vi "Maui 2.0. Set Subpanels.Config.vi"(6 "Append (F)":bool, 8 "error in":errorcluster, 9 "Section Cluster":variant, 10 "Path":path, 11 "Maui 2.0 in":refnum<class "Maui 2.0.lvclass">) -> (0 "error out":errorcluster, 1 "Found?":bool, 2 "Subpanels":refnum<class "SMO.lvclass">[](array[class]), 3 "Maui 2.0 out":refnum<class "Maui 2.0.lvclass">)   [LabVIEW 2019, in "Maui 2.0.lvclass"]
uses:
  Maui 2.0.lvclass
  Typedefs/Maui 2.0/Maui 2.0 Configuration.ctl
  <vilib>/Utility/config.llb/NI_LVConfig.lvlib
  <vilib>/JKI/JKI SMO/SMO/SMO.lvclass
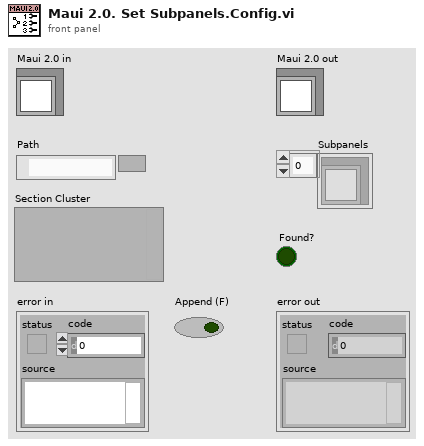
[diagram p1: front panel]
types:
  T1 = typedef "Maui 2.0.lvclass/Maui 2.0 Configuration.ctl" = cluster{"Paths":path[]}
  T2 = typedef "NI_LVConfig.lvlib/Config Data RefNum.ctl" = refnum<k1>
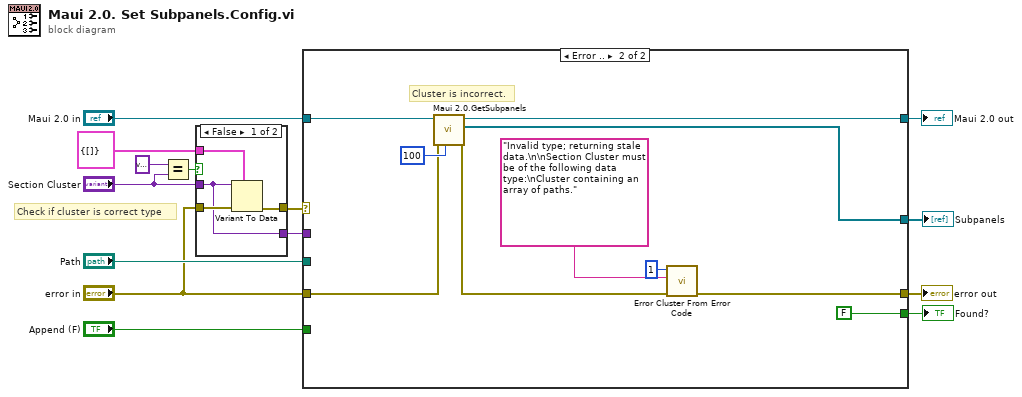
[diagram p0: block diagram]
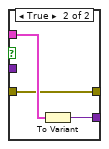
[diagram p2: hidden frame]
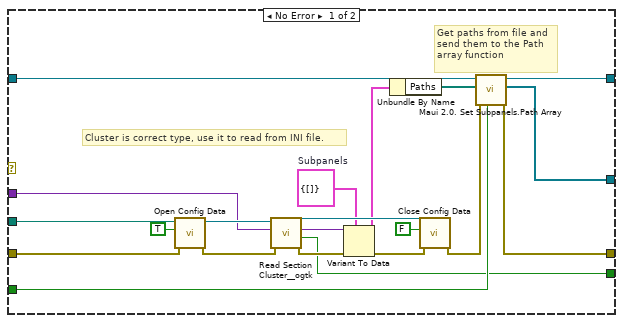
[diagram p3: hidden frame]
diagram:
  # "Check if cluster is correct type"
  n1 = Equal?(x=variant, y="Section Cluster") -> (x = y?=w3:bool)
  n2 = case shown="False" w3 {
    tunnel: T1 {"Paths"=[]} ("Subpanels") -> [w16 w21]
    tunnel: "Section Cluster" -> [w15 _]
    tunnel: [w18 w19] -> w6
    tunnel: "error in" -> [w17 w19]
    tunnel: [w15 w20] -> w5
    frame False {
      n3 = Variant To Data(error in=w17, type=w16, Variant=w15) -> (error out=w18:errorcluster)  [unwired: 1 out]
    }
    frame True {
      n4 = To Variant(anything=w21) -> (Variant=w20:variant)
    }
  }
  n5 = case shown="Error .." w6 {
    tunnel: "Path" -> [w42 _]
    tunnel: "error in" -> [w38 w43]
    tunnel: "Maui 2.0 in" -> [w32 w50]
    tunnel: [w31 w51] -> w12
    tunnel: [w29 w47] -> w11
    tunnel: "Append (F)" -> [w28 _]
    tunnel: [w25 w48] -> w9
    tunnel: [w24 FALSE ("all found?")] -> w8
    tunnel: w5 -> [w23 _]
    frame No Error {
      w22 = T1 {"Paths"=[]}  # Subpanels
      # "Get paths from file and send them to the Path array function"
      # "Cluster is correct type, use it to read from INI file."
      n6 = call <vilib>:"Open Config Data.vi"("error in (no error)"=w38, "create file if necessary (T)"=TRUE, "configuration file path"=w42) -> ("error out"=w37:errorcluster, "refnum"=w41:T2)  [unwired: 6 in, 1 out]
      n7 = call <userlib>:"Read Section Cluster__ogtk.vi"("error in (no error)"=w37, "Section Formatted Cluster Type"=w23, "refnum"=w41) -> ("error out"=w36:errorcluster, "all found?"=w24:bool, "Section Formatted Cluster"=w39:variant, "dup refnum"=w40:T2)  [unwired: 4 in, 1 out]
      n8 = Variant To Data(error in=w36, type=w22, Variant=w39) -> (data=w26:T1, error out=w35:errorcluster)
      n9 = Unbundle By Name(w26) -> ("Paths"=w27:path[])
      n10 = call <vilib>:"Close Config Data.vi"("error in (no error)"=w35, "write file if changed (T)"=FALSE, "refnum"=w40) -> ("error out"=w30:errorcluster)  [unwired: 7 in, 1 out]
      n11 = call-dynamic "Maui 2.0. Set Subpanels.Path Array.vi"("Append (F)"=w28, "error in (no error)"=w30, "Subpanel List"=w27, "Maui 2.0 in"=w32) -> ("error out"=w29:errorcluster, "Subpanels"=w25:refnum<class "SMO.lvclass">[], "Maui 2.0 out"=w31:refnum<class "Maui 2.0.lvclass">)  [unwired: 5 in]
    }
    frame Error {
      # "Cluster is incorrect."
      n12 = call "Maui 2.0.GetSubpanels.vi"("timeout in ms (-1)"=100, "error in (no error)"=w43, "Maui 2.0"=w50) -> ("error out"=w44:errorcluster, "Subpanels"=w48:refnum<class "SMO.lvclass">[], "Maui 2.0 out"=w51:refnum<class "Maui 2.0.lvclass">)  [unwired: 6 in]
      n13 = call <vilib>:"Error Cluster From Error Code.vi"("error in (no error)"=w44, "error message (\"\")"="Invalid type; returning stale data.\n\nSection Cluster must be of the following data type:\nCluster containing an array of paths." ("error message (\"\")"), "error code (0)"=1) -> ("error out"=w47:errorcluster)  [unwired: 6 in]
    }
  }
  "error out" <- w11
  "Maui 2.0 out" <- w12
  "Subpanels" <- w9
  "Found?" <- w8
